vi "Write Message Stream.vi"(10 "Message Stream":refnum<class "Message Stream.lvclass">, 11 "Cobra RT In":refnum<class "Cobra RT.lvclass">) -> (3 "Cobra RT Out":refnum<class "Cobra RT.lvclass">)   [LabVIEW 2019, in "Cobra RT.lvlib" / "Cobra RT.lvclass"]
uses:
  Cobra RT.lvclass
  <vilib>/ni/Actors/Network Endpoint Actors/Abstract Classes/Message Stream/Message Stream.lvclass
  Cobra RT.lvclass/Cobra RT.ctl
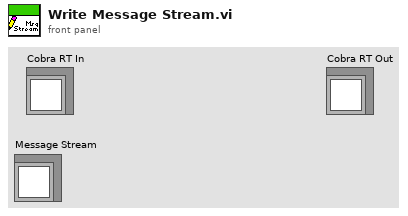
[diagram p1: front panel]
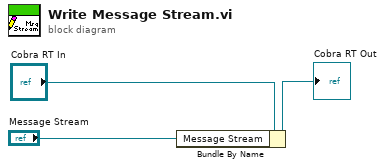
[diagram p0: block diagram]
diagram:
  n1 = Bundle By Name(cluster="Cobra RT In", "Message Stream"="Message Stream") -> (→"Cobra RT Out":refnum<class "Cobra RT.lvclass">)
